vi "Module Queue FGV.vi"(8 "error in":errorcluster, 10 "Queue Name":string, 11 "Action":T1=enum."Destroy") -> (0 "error out":errorcluster, 3 "Queue ref":refnum<queue>)   [LabVIEW 2018, in "Error Handler.lvlib"]
uses:
  Error Handler.lvlib
  ctl/Queue Actions.ctl
  ctl/Module Message.ctl
  ctl/Module State.ctl
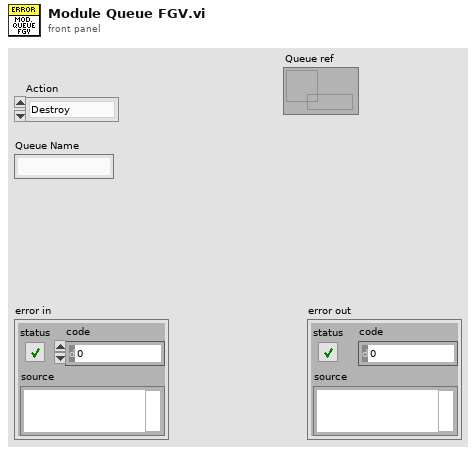
[diagram p1: front panel]
types:
  T1 = typedef "Error Handler.lvlib/Queue Actions.ctl" = enum16{"Create", "Get", "Destroy"}
  T2 = typedef "Error Handler.lvlib/Module Message.ctl" = cluster{"State":T3, "Data":variant}
  T3 = typedef "Error Handler.lvlib/Module State.ctl" = enum16{"Init", "Idle", "Error", "Close", "Handle External Error", "Log Error"}
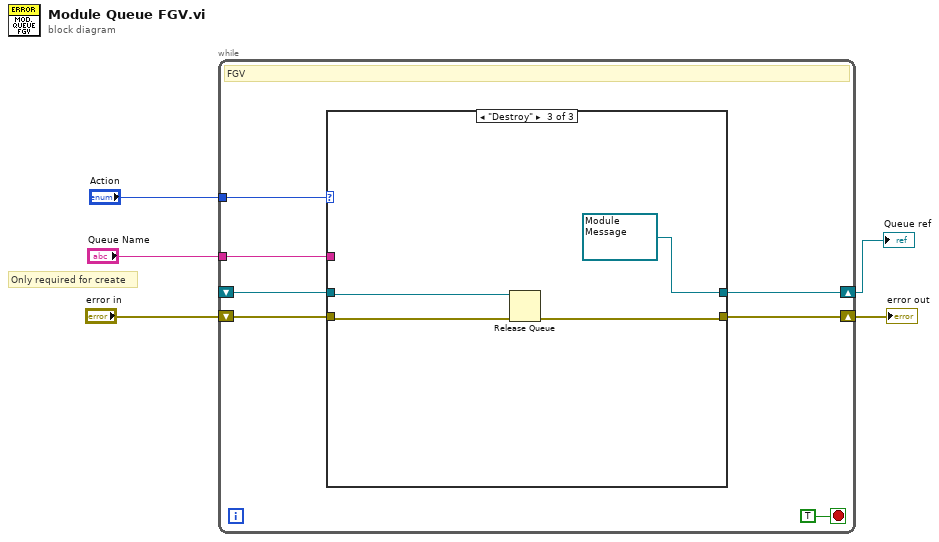
[diagram p0: block diagram]
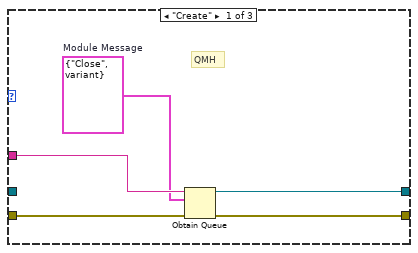
[diagram p2: hidden frame]
diagram:
  # "Only required for create"
  n1 = while {
    tunnel: "Action" -> [w12]
    shift-right: [w9] -> w4
    shift-left: "error in" -> [w8]
    shift-right: [w10] -> w1
    shift-left: _ -> [w7]
    tunnel: "Queue Name" -> [w6]
    stop <- TRUE stop-if-true
    # "FGV"
    n2 = case shown="\"Destroy\"" w12 {
      tunnel: [w17 w19 refnum<queue> refnum ("queue out")] -> w10
      tunnel: [w16 w18 w21] -> w9
      tunnel: w8 -> [w15 w18 w22]
      tunnel: w7 -> [_ w19 w23]
      tunnel: w6 -> [w14 _ _]
      frame "Create" {
        w13 = T2 {"State"=enum."Close", "Data"=variant}  # Module Message
        # "QMH"
        n3 = Obtain Queue(name (unnamed)=w14, element data type=w13, error in (no error)=w15) -> (queue out=w17:refnum<queue>, error out=w16:errorcluster)  [unwired: 2 in, 1 out]
      }
      frame "Get", Default {
      }
      frame "Destroy" {
        n4 = Release Queue(queue=w23, error in (no error)=w22) -> (error out=w21:errorcluster)  [unwired: 1 in, 2 out]
      }
    }
  }
  "error out" <- w4
  "Queue ref" <- w1
